vi "Launch Root Error Reporter Actor.vi"(4 "Debug Alias":string, 6 "Open Actor Core front panel? (F)":bool, 8 "error in (no error)":errorcluster, 9 "Error Manager in":refnum<class "Error Manager.lvclass">, 10 "Error Reporter in":refnum<class "Error Reporter.lvclass">) -> (0 "error out":errorcluster, 2 "Actor's Enqueuer":refnum<class "Message Enqueuer.lvclass">)   [LabVIEW 2024, in "Error Reporting Actor.lvlib" / "Error Reporter.lvlib" / "Error Reporter.lvclass"]
uses:
  Error Reporter.lvclass
  C:/Program Files (x86)/National Instruments/LabVIEW 2024/vi.lib/ActorFramework/Actor/Actor.lvclass
  <vilib>/ActorFramework/Message Enqueuer/Message Enqueuer.lvclass
  Error Manager/Error Manager/Error Manager.lvclass
  Error Reporter.lvclass/Error Reporter.ctl
  <vilib>/ActorFramework/Actor/Actor.lvclass
  C:/Users/uspoaotto/OneDrive - Oregon Tool/Desktop/working copies/errorReportingActor/src/Error Reporting Actor/Error Manager/Error Manager/Error Manager.lvclass
  C:/Users/uspoaotto/OneDrive - Oregon Tool/Desktop/working copies/errorReportingActor/src/Error Reporting Actor/~Error/~Error/~Error.lvclass
  C:/Users/uspoaotto/OneDrive - Oregon Tool/Desktop/working copies/errorReportingActor/src/Error Reporting Actor/Error Reporter/Error Reporter/Error Reporter.lvclass
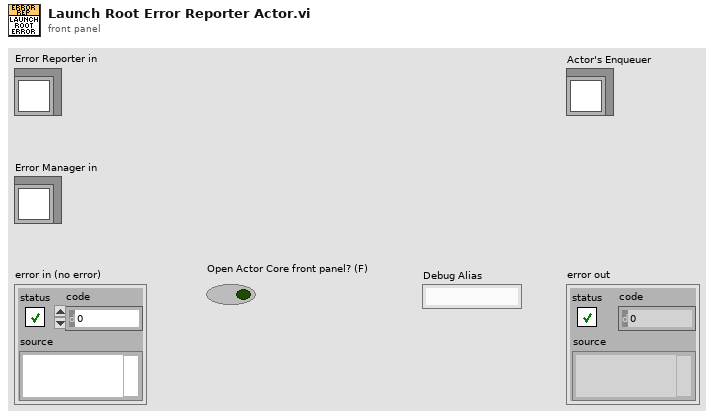
[diagram p1: front panel]
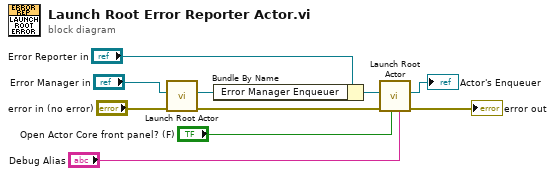
[diagram p0: block diagram]
diagram:
  n1 = call <vilib>:"Launch Root Actor.vi"("error in (no error)"="error in (no error)", "Actor"="Error Manager in") -> ("error out"=w6:errorcluster, "Actor's Enqueuer"=w4:refnum<class "Message Enqueuer.lvclass">)  [unwired: 8 in]
  n2 = Bundle By Name(cluster="Error Reporter in", "Error Manager Enqueuer"=w4) -> (w3:refnum<class "Error Reporter.lvclass">)
  n3 = call <vilib>:"Launch Root Actor.vi"("Debug Alias"="Debug Alias", "Open Actor Core front panel? (F)"="Open Actor Core front panel? (F)", "error in (no error)"=w6, "Actor"=w3) -> ("error out"=→"error out":errorcluster, "Actor's Enqueuer"=→"Actor's Enqueuer":refnum<class "Message Enqueuer.lvclass">)  [unwired: 6 in]
